vi "testPersistentData.vi"() -> ()   [LabVIEW 2017, in "Theory.Tests.lvlib"]
uses:
  Theory.Tests.lvlib
  ControlData.ctl
  Theory/Theory.lvclass
  Support/Support.lvlib
  Assertion/Assertion.lvlib
panel:
  out "error out":errorcluster
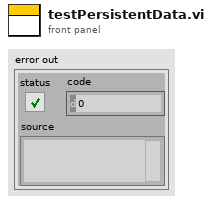
[diagram p1: front panel]
types:
  T1 = typedef "ControlData.ctl" = cluster{"Name":string, "Data":variant}
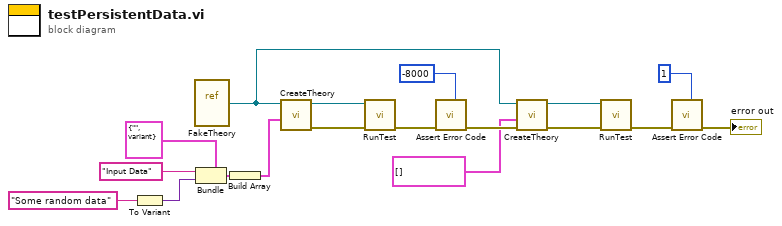
[diagram p0: block diagram]
diagram:
  n1 = To Variant(anything="Some random data" ("key")) -> (Variant=w12:variant)
  n2 = vi-ref "FakeTheory.vi"() -> (w3:refnum<vi>)
  n3 = Bundle(cluster=T1 {"Name"="", "Data"=variant} ("Control Data"), "Name"="Input Data" ("key"), "Data"=w12) -> (w13:T1)
  n4 = Build Array(w13) -> (w1:T1[])
  n5 = call "CreateTheory.vi"("Control Data"=w1, "VI Refnum"=w3) -> ("error out"=w17:errorcluster, "Theory"=w18:refnum<class "Theory.lvclass">)  [unwired: 8 in]
  n6 = call-dynamic "RunTest.vi"("error in (no error)"=w17, "Theory in"=w18) -> ("error out"=w16:errorcluster)  [unwired: 8 in, 1 out]
  n7 = call "Assert Error Code.vi"("Expected"=-8000, "error in (no error)"=w16) -> ("error out"=w8:errorcluster)  [unwired: 9 in]
  n8 = call "CreateTheory.vi"("error in (no error)"=w8, "Control Data"=T1[] [] ("Array"), "VI Refnum"=w3) -> ("error out"=w10:errorcluster, "Theory"=w9:refnum<class "Theory.lvclass">)  [unwired: 7 in]
  n9 = call-dynamic "RunTest.vi"("error in (no error)"=w10, "Theory in"=w9) -> ("error out"=w7:errorcluster)  [unwired: 8 in, 1 out]
  n10 = call "Assert Error Code.vi"("Expected"=1, "error in (no error)"=w7) -> ("error out"=→"error out":errorcluster)  [unwired: 9 in]
